vi "AD5781ValidVoltCheck.vi"(4 "U32":u32 format="%024b") -> (1 "coerced(x)":u32 format="%024b")   [LabVIEW 2014]
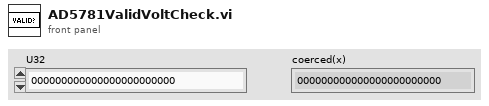
[diagram p1: front panel]
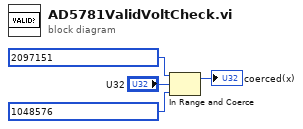
[diagram p0: block diagram]
diagram:
  n1 = In Range and Coerce(upper limit=u32 2097151 ("lower limit"), x="U32", lower limit=u32 1048576) -> (coerced(x)=→"coerced(x)":u32)  [unwired: 1 out]
